vi "CRYProject Editor Init.vi"   [LabVIEW 2013]
uses:
  CRYSystem/Typedef Control/CRYTS.ctl
  CRYSystem/Typedef Control/CRYStep.ctl
  CRYProject Editor Global.vi
  CRYMainGlobal.vi
  CRYSystem/Calibration/SubVI/CRYCal Global.vi
  CRYSystem/Task Sequence/CRYProject Run Control Global.vi
panel:
  # "Project Init.\nconfiguration recent file and so on."
types:
  T1 = typedef "CRYTS.ctl" = cluster{"No.TS":u16, "TS File Path":path, "TS Name":string, "EditStepName":string, "Steps":T2[], "New State":bool, "Change State":bool, "Flattened CurveLib Data":string, "Document Data":string, "EditStepNo":u16, "Operator Start File":string, "Sequence Type":string, "Sequence Language":string}
  T2 = typedef "CRYStep.ctl" = cluster{"No.VI":i32, "Category":string, "StepName":string, "Seq setup flattened":string, "Comment":string, "Steps config.":bool[], "Jump config":i32[], "Start":dbl, "Increment":dbl, "Name":string, "Unit":string, "Y data":u16, "Y prefix":string, "Y dB ref":dbl, "Y unit":string, "Repeat State Array":cluster{"Start":dbl, "Increment":dbl, "Count":i32, "Num":i32}[]}
  T3 = enum32{"English", "Chinese", "Korean", "Japanese", "Russian", "Chinese traditional"}
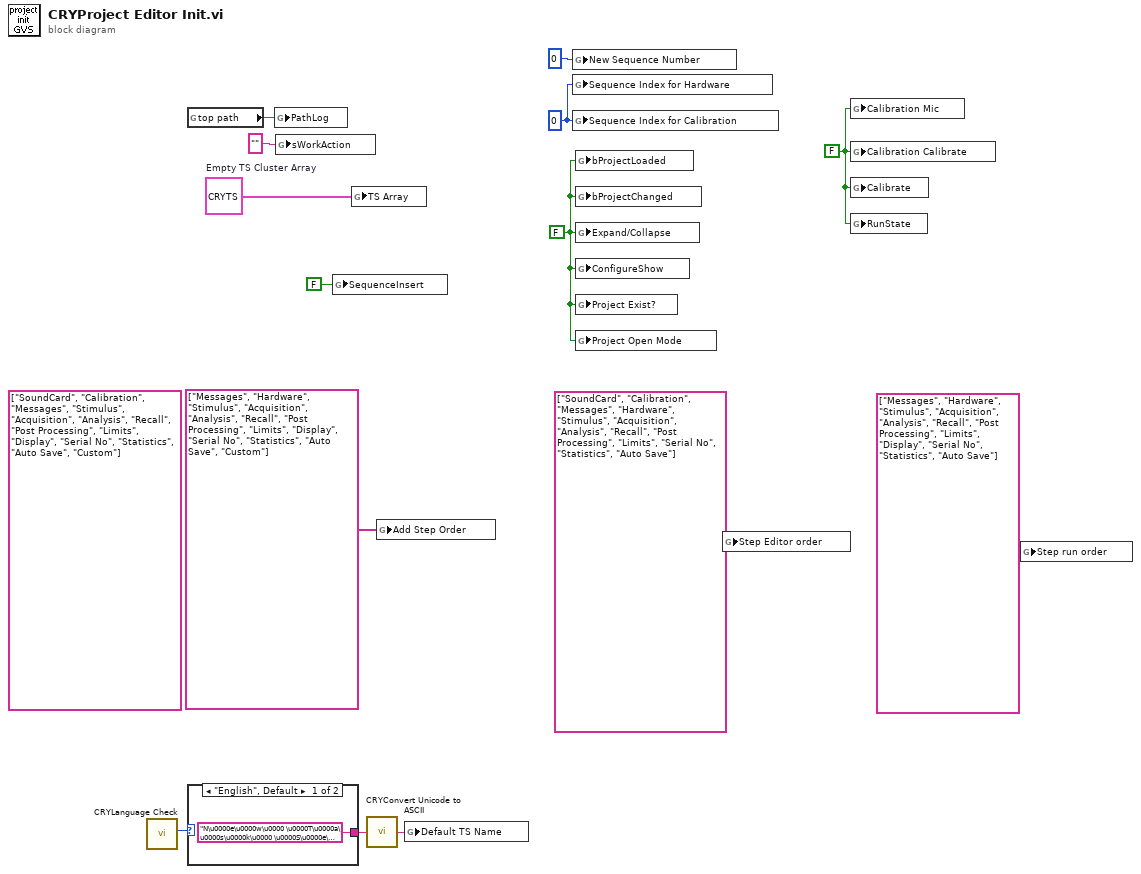
[diagram p0: block diagram]
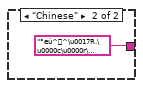
[diagram p2: hidden frame]
diagram:
  (unwired) string[] ["SoundCard", "Calibration", "Messages", "Stimulus", "Acquisition", "Analysis", "Recall", "Post Processing", "Limits", "Display", "Serial No", "Statistics", "Auto Save", "Custom"] ("Add Step Order")
  w5 = FALSE ("Calibrate")
  w10 = 0 ("Sequence Index for Hardware")
  w6 = FALSE ("Project Exist?")
  w14 = T1 {"No.TS"=0, "TS File Path"=path "", "TS Name"="", "EditStepName"="", "Steps"=[], "New State"=FALSE, "Change State"=FALSE, "Flattened CurveLib Data"="", "Document Data"="", "EditStepNo"=0, "Operator Start File"="", "Sequence Type"="", "Sequence Language"=""}  # Empty TS Cluster Array
  n1 = call "CRYLanguage Check.vi"() -> ("Language"=w2:T3)  [unwired: 10 in, 1 out]
  n2 = global read "CRYMainGlobal.vi" "top path"() -> (w12:path)
  n3 = case shown="\"English\", Default" w2 {
    tunnel: ["N\u0000e\u0000w\u0000 \u0000T\u0000a\u0000s\u0000k\u0000 \u0000S\u0000e\u0000q\u0000u\u0000e\u0000n\u0000c\u0000e\u0000.\u0000c\u0000r\u0000y\u0000" ("Default TS Name") "°eú^^\u0017R.\u0000c\u0000r\u0000y\u0000" ("Default TS Name")] -> w3
    frame "English", Default {
    }
    frame "Chinese" {
    }
  }
  n4 = global write "CRYProject Editor Global.vi" "PathLog"(w12) -> ()
  n5 = global write "CRYProject Editor Global.vi" "sWorkAction"("" ("sWorkAction")) -> ()
  n6 = global write "CRYProject Editor Global.vi" "SequenceInsert"(FALSE ("SequenceInsert")) -> ()
  n7 = global write "CRYProject Editor Global.vi" "TS Array"(w14) -> ()
  n8 = call "CRYConvert Unicode to ASCII.vi"("Unicode"=w3) -> ("ASCII"=w1:string)  [unwired: 4 in]
  n9 = global write "CRYMainGlobal.vi" "Add Step Order"(string[] ["Messages", "Hardware", "Stimulus", "Acquisition", "Analysis", "Recall", "Post Processing", "Limits", "Display", "Serial No", "Statistics", "Auto Save", "Custom"] ("Add Step Order")) -> ()
  n10 = global write "CRYProject Editor Global.vi" "Default TS Name"(w1) -> ()
  n11 = global write "CRYProject Editor Global.vi" "New Sequence Number"(u16 0 ("New Sequence Number")) -> ()
  n12 = global write "CRYProject Editor Global.vi" "Sequence Index for Hardware"(w10) -> ()
  n13 = global write "CRYProject Editor Global.vi" "Sequence Index for Calibration"(w10) -> ()
  n14 = global write "CRYProject Editor Global.vi" "bProjectLoaded"(w6) -> ()
  n15 = global write "CRYProject Editor Global.vi" "bProjectChanged"(w6) -> ()
  n16 = global write "CRYProject Editor Global.vi" "Expand/Collapse"(w6) -> ()
  n17 = global write "CRYProject Editor Global.vi" "ConfigureShow"(w6) -> ()
  n18 = global write "CRYProject Editor Global.vi" "Project Exist?"(w6) -> ()
  n19 = global write "CRYProject Editor Global.vi" "Project Open Mode"(w6) -> ()
  n20 = global write "CRYMainGlobal.vi" "Step Editor order"(string[] ["SoundCard", "Calibration", "Messages", "Hardware", "Stimulus", "Acquisition", "Analysis", "Recall", "Post Processing", "Limits", "Serial No", "Statistics", "Auto Save"] ("Step Editor order")) -> ()
  n21 = global write "CRYCal Global.vi" "Calibration Mic"(w5) -> ()
  n22 = global write "CRYCal Global.vi" "Calibration Calibrate"(w5) -> ()
  n23 = global write "CRYCal Global.vi" "Calibrate"(w5) -> ()
  n24 = global write "CRYProject Run Control Global.vi" "RunState"(w5) -> ()
  n25 = global write "CRYMainGlobal.vi" "Step run order"(string[] ["Messages", "Hardware", "Stimulus", "Acquisition", "Analysis", "Recall", "Post Processing", "Limits", "Display", "Serial No", "Statistics", "Auto Save"] ("Step run order")) -> ()
